vi "Get Template Path.vi"(11 "Abstract Message Scripter in":refnum<class "Abstract Message Scripter.lvclass">) -> (2 "Template Path":path)   [LabVIEW 2020, in "Message Maker.lvlib" / "Abstract Message Scripter.lvclass"]
uses:
  Abstract Message Scripter.lvclass
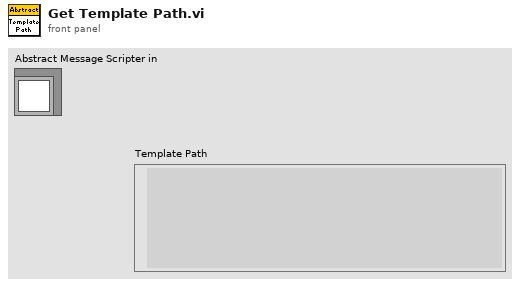
[diagram p1: front panel]
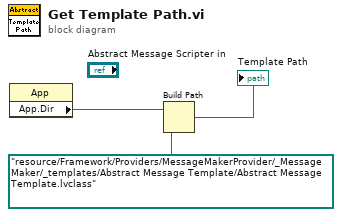
[diagram p0: block diagram]
diagram:
  n1 = property class="App"() -> ("App.Dir"=w1:path)  [unwired: 2 in, 2 out]
  n2 = Build Path(base path=w1, name or relative path=path "resource/Framework/Providers/MessageMakerProvider/_Message Maker/_templates/Abstract Message Template/Abstract Message Template.lvclass" ("Template Path")) -> (appended path=→"Template Path":path)
